vi "Distance of 2 Points.vi"(0 "X [Pixels]":dbl, 1 "Y [Pixels]":dbl, 2 "X of point [Pixels]":dbl, 3 "Y of point [Pixels]":dbl, 4 "Conversion ratio (X*pixels = 1 * inch)":dbl) -> (5 "Distance on ground [Meters]":dbl, 6 "Distance on ground [Inches]":dbl)   [LabVIEW 2012]
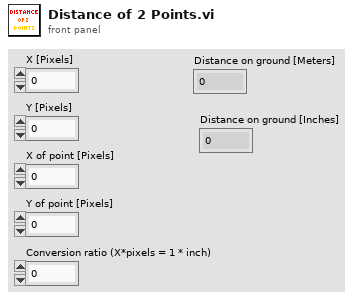
[diagram p1: front panel]
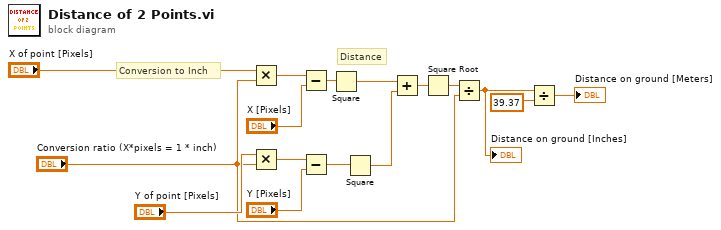
[diagram p0: block diagram]
diagram:
  # "Distance"
  # "Conversion to Inch"
  n1 = Multiply(x="X of point [Pixels]", y="Conversion ratio (X*pixels = 1 * inch)") -> (x*y=w10:dbl)
  n2 = Multiply(x="Y of point [Pixels]", y="Conversion ratio (X*pixels = 1 * inch)") -> (x*y=w8:dbl)
  n3 = Subtract(x=w10, y="X [Pixels]") -> (x-y=w12:dbl)
  n4 = Subtract(x=w8, y="Y [Pixels]") -> (x-y=w16:dbl)
  n5 = Square(x=w12) -> (x^2=w13:dbl)
  n6 = Square(x=w16) -> (x^2=w14:dbl)
  n7 = Add(x=w13, y=w14) -> (x+y=w15:dbl)
  n8 = Square Root(x=w15) -> (sqrt(x)=w3:dbl)
  n9 = Divide(x=w3, y="Conversion ratio (X*pixels = 1 * inch)") -> (x/y=w1:dbl)
  "Distance on ground [Inches]" <- w1
  n10 = Divide(x=w1, y=39.37) -> (x/y=→"Distance on ground [Meters]":dbl)
